vi "Get All CD Item Property Values.vi"(8 "error in (no error)":errorcluster, 11 "CD Parameter Manager in":refnum<class "CD Parameter Manager.lvclass">) -> (0 "error out":errorcluster, 3 "CD Parameter Manager out":refnum<class "CD Parameter Manager.lvclass">)   [LabVIEW 2019, in "CD Parameter Manager API.lvlib" / "CD Parameter Manager.lvclass"]
uses:
  CD Parameter Manager.lvclass
  CD Parameter Manager.lvclass/CD Parameter Manager.ctl
  Parameter Class/Parameter.lvclass
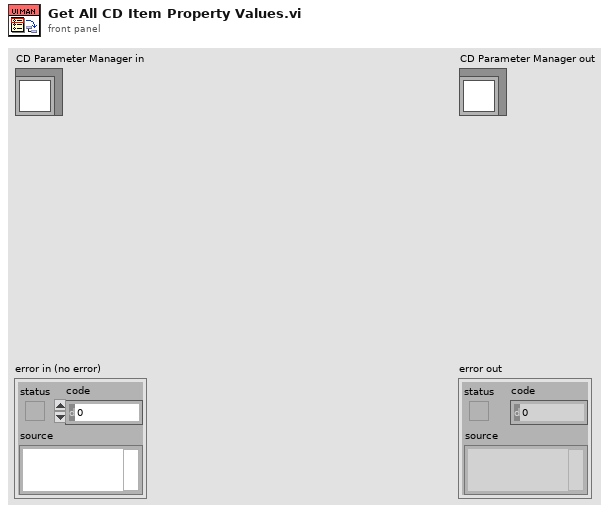
[diagram p1: front panel]
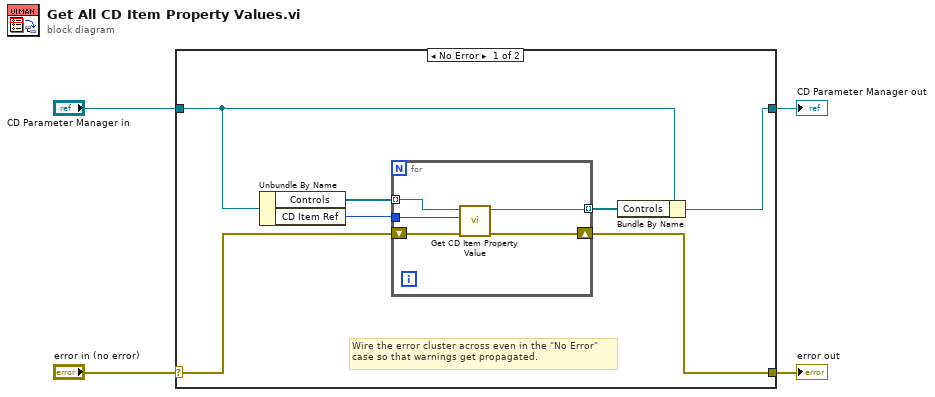
[diagram p0: block diagram]
diagram:
  n1 = case shown="No Error" "error in (no error)" {
    selector: "error in (no error)" -> [w10 w18]
    tunnel: [w5 w18] -> w3
    tunnel: [w6 w17] -> w1
    tunnel: "CD Parameter Manager in" -> [w7 w17]
    frame No Error {
      # "Wire the error cluster across even in the \"No Error\"\ncase so that warnings get propagated."
      n2 = Unbundle By Name(w7) -> ("Controls"=w11:refnum<class "Parameter.lvclass">[], "CD Item Ref"=w9:u64)
      n3 = for {
        tunnel: w9 -> [w15]
        tunnel: w11 -> [w14] mode=indexing
        shift-right: [w13] -> w5
        shift-left: w10 -> [w16]
        tunnel: [w12] -> w8 mode=indexing
        n4 = call-dynamic "Get CD Item Property Value.vi"("error in (no error)"=w16, "CD Item Ref in"=w15, "Parameter in"=w14) -> ("error out"=w13:errorcluster, "Parameter out"=w12:refnum<class "Parameter.lvclass">)  [unwired: 7 in]
      }
      n5 = Bundle By Name(cluster=w7, "Controls"=w8) -> (w6:refnum<class "CD Parameter Manager.lvclass">)
    }
    frame Error {
    }
  }
  "error out" <- w3
  "CD Parameter Manager out" <- w1
